vi "TagDB Refmgr-Remove.vi"(8 "error in (no error)":errorcluster, 11 "TagDB in":T1) -> (0 "error out":errorcluster, 1 "Keys":string[](array[string]), 2 "References":refnum<vi>[](array[refnum]), 3 "TagDB out":T1)   [LabVIEW 2017, in "TagDB RefManager.lvlib"]
uses:
  TagDB RefManager.lvlib
  <userlib>/_NEVSTOP/TagDB/Typedef/TagDB.ctl
  9d601a23-f96e-4540-83e7-41ff60b3d226.vi
  <userlib>/_NEVSTOP/TagDB/_Support/Error/_Clear Errors.vi
  9d601a23-f96e-4540-83e7-41ff60b3d226.vi/29b2ea6d-6d7f-4e4a-ad31-a5cb760462c7.vi
  <userlib>/_NEVSTOP/TagDB/API/TagDB-Status.vi
  <userlib>/_NEVSTOP/TagDB/_Support/DataAccess/_NameCacher.vi
  <userlib>/_NEVSTOP/TagDB/_Support/Error/_[error50001]Can't Found Value.vi
  <userlib>/_NEVSTOP/TagDB/_Support/Change Detector/TagDB dbChanged.vi
  <userlib>/_NEVSTOP/TagDB/_Support/DataAccess/TagDB Ref to DVR.vi
  <userlib>/_NEVSTOP/TagDB/_Support/Error/_[error50000]Invalid DB REF.vi
  <userlib>/_NEVSTOP/TagDB/_Support/URL/TRIM-BOTH-SPACE.vi
  <userlib>/_NEVSTOP/TagDB/_Support/Error/_[error50002]Invalid DataType.vi
  <vilib>/Utility/error.llb/Trim Whitespace.vi
  <userlib>/_NEVSTOP/TagDB/_Support/Error/_Build Error Cluster.vi
  <userlib>/_NEVSTOP/TagDB/TagDB.lvlib
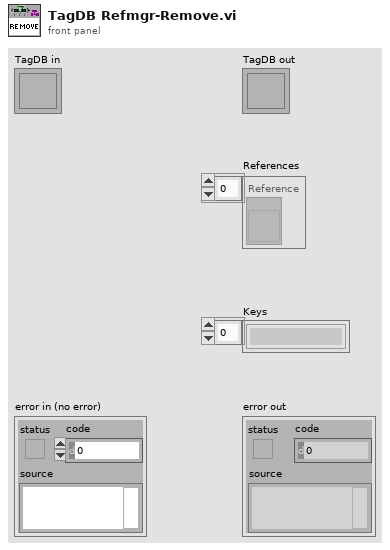
[diagram p1: front panel]
types:
  T1 = typedef "TagDB.lvlib/TagDB.ctl" = refnum<k1>
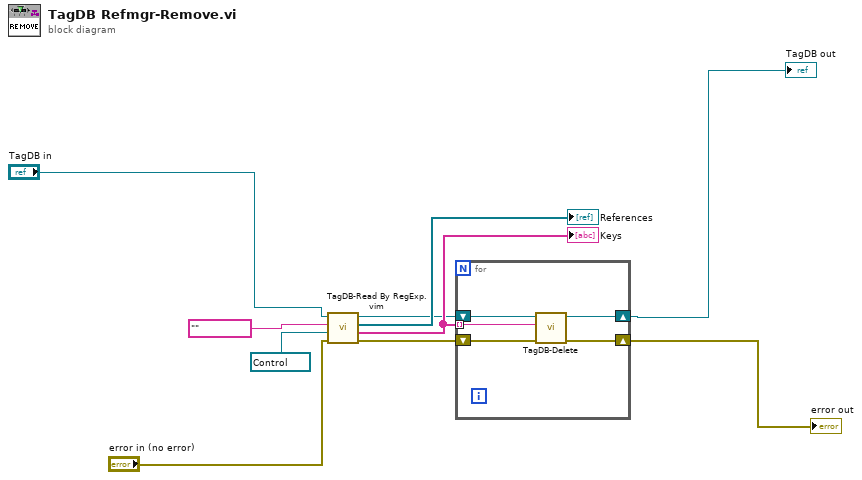
[diagram p0: block diagram]
diagram:
  n1 = call "TagDB-Read By RegExp.vim"("error in (no error)"="error in (no error)", "Type"=refnum<vi> refnum, "RegExp"="", "DB Ref"="TagDB in") -> ("error out"=w5:errorcluster, "names"=w8:string[], "value"=→"References":refnum<vi>[], "DB Ref(dup)"=w6:T1)  [unwired: 4 in]
  "Keys" <- w8
  n2 = for {
    tunnel: w8 -> [w11] mode=indexing
    shift-right: [w14] -> w3
    shift-left: w6 -> [w15]
    shift-right: [w13] -> w2
    shift-left: w5 -> [w12]
    n3 = call <userlib>:"TagDB-Delete.vi"("error in (no error)"=w12, "name"=w11, "TagDB"=w15) -> ("error out"=w13:errorcluster, "TagDB(dup)"=w14:T1)  [unwired: 7 in]
  }
  "error out" <- w2
  "TagDB out" <- w3
